vi "sv_UFF58 Write Ordinate Data.vi"(0 "function refnum":refnum<k20>, 1 "channel to write":enum16{"X", "Y Real", "Y Imaginary"}(ring)=enum."Y Real", 5 "ordinate channel name":string="Yimag", 9 "ordinate data":dbl[](array[numeric]), 11 "error in (no error)":errorcluster) -> (4 "dup function refnum":refnum<k20>, 15 "error out":errorcluster)   [LabVIEW 2017, in "SoundVib_UFF58.lvlib"]
doc: "This VI writes the <B>ordinate data</B> for the given <B>channel to write</B> in the input <B>function refnum</B>"
uses:
  <vilib>/addons/Sound and Vibration/svt_UFF58/SoundVib_UFF58.lvlib
  <vilib>/Platform/storage/Storage.llb/Get Property (Storage Refnums).vi
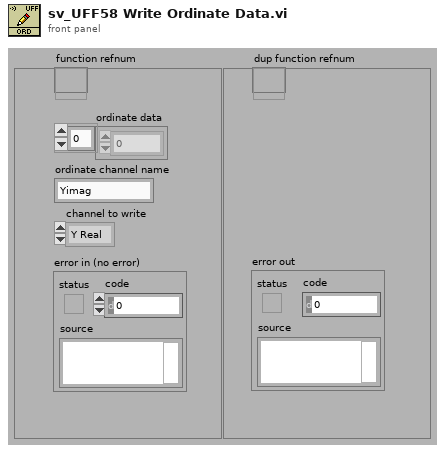
[diagram p1: front panel]
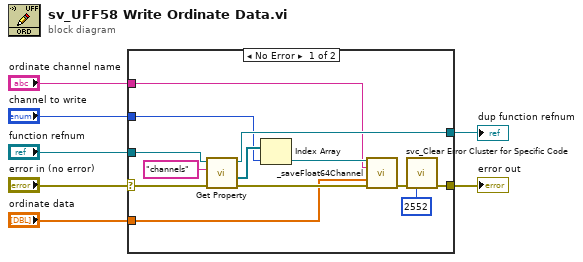
[diagram p0: block diagram]
diagram:
  n1 = case shown="No Error" "error in (no error)" {
    selector: "error in (no error)" -> [w14 w21]
    tunnel: "ordinate data" -> [w13 _]
    tunnel: [w11 w21] -> w6
    tunnel: "function refnum" -> [w18 w22]
    tunnel: [w15 w22] -> w2
    tunnel: "channel to write" -> [w9 _]
    tunnel: "ordinate channel name" -> [w8 _]
    frame No Error {
      n2 = call-poly <vilib>:"Get Property.vi"("error in (no error)"=w14, "Property name"="channels", "storage refnum"=w18) -> ("error out"=w17:errorcluster, "Value"=w20:refnum<k20>[], "storage refnum out"=w15:refnum<k20>)  [unwired: 6 in]
      n3 = Index Array(array=w20, index=w9) -> (element=w16:refnum<k20>)
      n4 = call <vilib>:"_saveFloat64Channel.vi"("Data object in"=w16, "Name"=w8, "Values"=w13, "error in (no error)"=w17) -> ("error out"=w12:errorcluster)  [unwired: 9 in, 2 out]
      n5 = call <vilib>:"svc_Clear Error Cluster for Specific Code.vi"("error in (no error)"=w12, "code"=2552 ("warning code")) -> ("error out"=w11:errorcluster)  [unwired: 12 in, 1 out]
    }
    frame Error {
    }
  }
  "error out" <- w6
  "dup function refnum" <- w2
